vi "SALS.vi"() -> ()   [LabVIEW 2024]
uses:
  <vilib>/vision/driver/NI_Vision_Acquisition_Software.lvlib
  <vilib>/vision/driver/IMAQdx.llb/IMAQdx Camera Control Mode.ctl
  <vilib>/DAQmx/create/channels.llb/DAQmx Create Channel (AI-Voltage-Basic).vi
panel:
  in  "Pixel Size (µm)":dbl
  in  "Sample Height (mm)":dbl
  in  "Sample Width (mm)":dbl
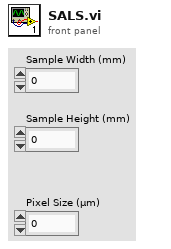
[diagram p1: front panel]
types:
  T1 = enum16{"Setup", "Configure", "Move", "Capture", "Finish"}
  T2 = typedef "NI_Vision_Acquisition_Software.lvlib/IMAQdx Camera Control Mode.ctl" = enum32{"Controller", "Listener"}
  T3 = typedef "Image Type" = u32
  T4 = typedef "IMAQ Image.ctl" = refnum<image>
  T5 = typedef "IMAQdx.ctl" = refnum<k21>
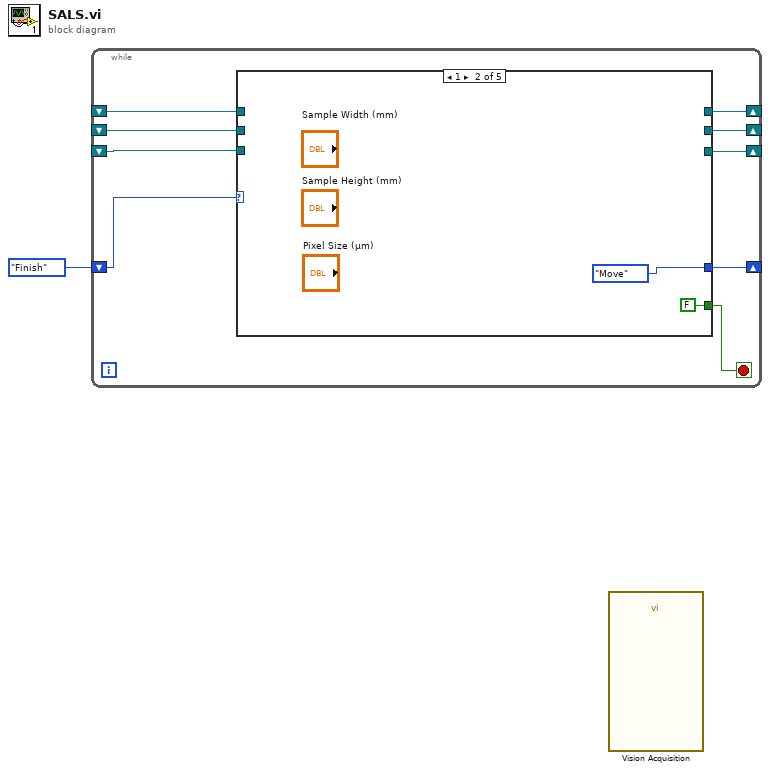
[diagram p0: block diagram]
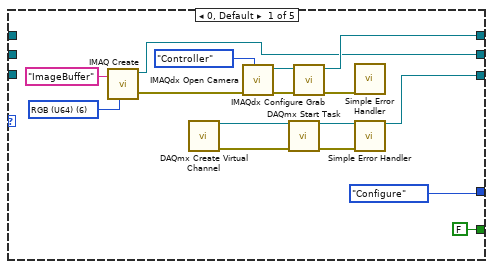
[diagram p2: hidden frame]
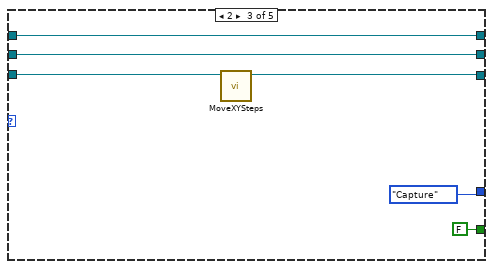
[diagram p3: hidden frame]
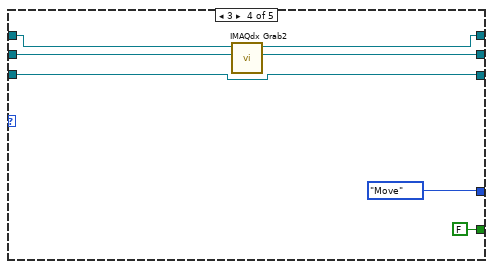
[diagram p4: hidden frame]
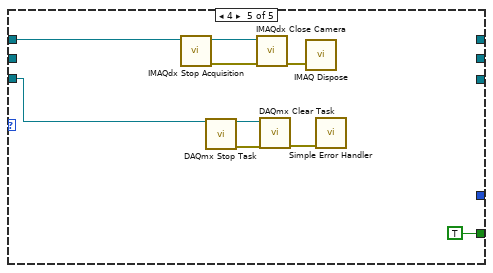
[diagram p5: hidden frame]
diagram:
  n1 = while {
    shift-right: [w8] -> _
    shift-left: _ -> [w3]
    shift-right: [w9] -> _
    shift-left: _ -> [w4]
    shift-right: [w10] -> _
    shift-left: _ -> [w5]
    shift-right: [w7] -> _
    shift-left: T1."Finish" -> [w6]
    stop <- w2 stop-if-true
    n2 = case shown="1" w6 {
      tunnel: [w18 _ w30 w36 _] -> w8
      tunnel: [w17 _ w31 w38 _] -> w9
      tunnel: [w14 _ w32 w37 _] -> w10
      tunnel: [T1."Configure" T1."Move" T1."Capture" enum16{"Move"}."Move" _] -> w7
      tunnel: w5 -> [_ _ w32 w39 _]
      tunnel: w4 -> [_ _ w31 w40 w45]
      tunnel: w3 -> [_ _ w33 w36 w44]
      tunnel: [FALSE FALSE FALSE FALSE TRUE] -> w2
      frame 0, Default {
        w15 = T3 6 items=["Grayscale (U8)", "Grayscale (I16)", "Grayscale (SGL)", "Complex (CSG)", "RGB (U32)", "HSL (U32)", "RGB (U64)", "Grayscale (U16)"] ("Image Type")
        n3 = call "IMAQ Create"("Image Name"="ImageBuffer", "Image Type"=w15) -> ("New Image"=w14:T4, "error out"=w23:errorcluster)  [unwired: 3 in]
        n4 = call-poly <vilib>:"DAQmx Create Virtual Channel.vi"() -> ("task out"=w19:refnum<k21>, "error out"=w20:errorcluster)  [unwired: 14 in]
        n5 = call <vilib>:"IMAQdx Open Camera.vi"("Camera Control Mode"=IMAQdx_Camera_Control_Mode."Controller", "error in"=w23) -> ("error out"=w24:errorcluster, "Session Out"=w25:T5)  [unwired: 8 in]
        n6 = call <vilib>:"DAQmx Start Task.vi"("task/channels in"=w19, "error in"=w20) -> ("task out"=w18:refnum<k21>, "error out"=w21:errorcluster)  [unwired: 12 in]
        n7 = call <vilib>:"IMAQdx Configure Grab.vi"("error in"=w24, "Session In"=w25) -> ("error out"=w22:errorcluster, "Session Out"=w17:T5)  [unwired: 8 in]
        n8 = call <vilib>:"Simple Error Handler.vi"("error in (no error)"=w22) -> ()  [unwired: 4 in, 5 out]
        n9 = call <vilib>:"Simple Error Handler.vi"("error in (no error)"=w21) -> ()  [unwired: 4 in, 5 out]
      }
      frame 1 {
      }
      frame 2 {
        n10 = call "MoveXYSteps.vi"("task in"=w33) -> ("task out"=w30:refnum<k21>)  [unwired: 10 in]
      }
      frame 3 {
        n11 = call <vilib>:"IMAQdx Grab2.vi"("Image In"=w39, "Session In"=w40) -> ("Image Out"=w37:T4, "Session Out"=w38:T5)  [unwired: 6 in, 2 out]
      }
      frame 4 {
        n12 = call <vilib>:"IMAQdx Stop Acquisition.vi"("Session In"=w45) -> ("error out"=w47:errorcluster, "Session Out"=w48:T5)  [unwired: 9 in]
        n13 = call <vilib>:"DAQmx Stop Task.vi"("task/channels in"=w44) -> ("task out"=w43:refnum<k21>, "error out"=w42:errorcluster)  [unwired: 13 in]
        n14 = call <vilib>:"IMAQdx Close Camera.vi"("error in"=w47, "Session In"=w48) -> ("error out"=w49:errorcluster)  [unwired: 9 in]
        n15 = call <vilib>:"DAQmx Clear Task.vi"("task in"=w43, "error in"=w42) -> ("error out"=w41:errorcluster)  [unwired: 13 in]
        n16 = call "IMAQ Dispose"("error in (no error)"=w49) -> ()  [unwired: 5 in, 1 out]
        n17 = call <vilib>:"Simple Error Handler.vi"("error in (no error)"=w41) -> ()  [unwired: 4 in, 5 out]
      }
    }
  }
  n18 = call "Vision Acquisition"() -> ()  [unwired: 26 in, 2 out]
